vi "TIFF camera test 3.vi"(8 "Gain":i32=100 min=100 max=2000 step=1, 9 "Exposure time (ms)":dbl=100.0 min=1.0 max=10000.0 step=1.0) -> (2 "Image out":T1(plugin-control))   [LabVIEW 2017]
uses:
  libtiff/ctiff.llb/__CTIFFNewFileAndStyleUINT16.vi
  libtiff/ctiff.llb/__CTIFFAddNewPageUINT16.vi
panel:
  out "Saving":bool
  in  "delay (ms)":dbl=100.0 min=0.0 max=2000.0 step=1.0
  in  "#-frames":i32=100 min=0 max=2000 step=1
  out "Capturing":bool
  in  "TIF file path":path=path "C:/Users/Chip Scope/Desktop/test.tif"
  in  "stop":bool
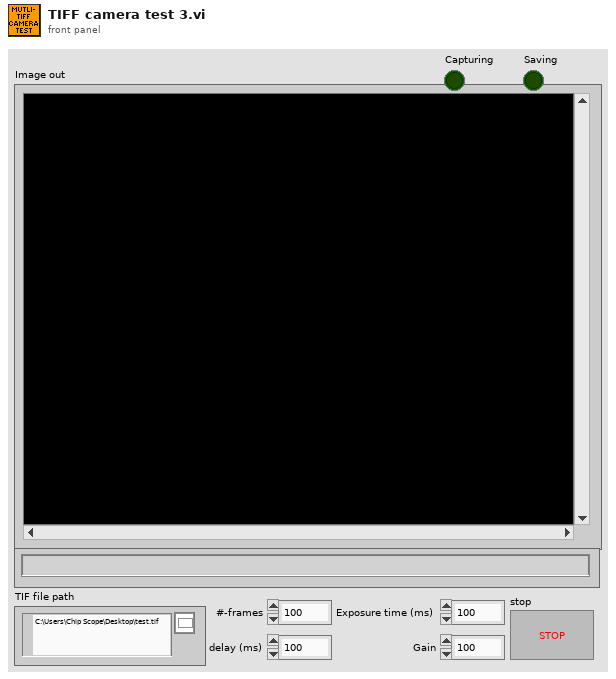
[diagram p1: front panel]
types:
  T1 = typedef "IMAQ Image.ctl" = refnum<image>
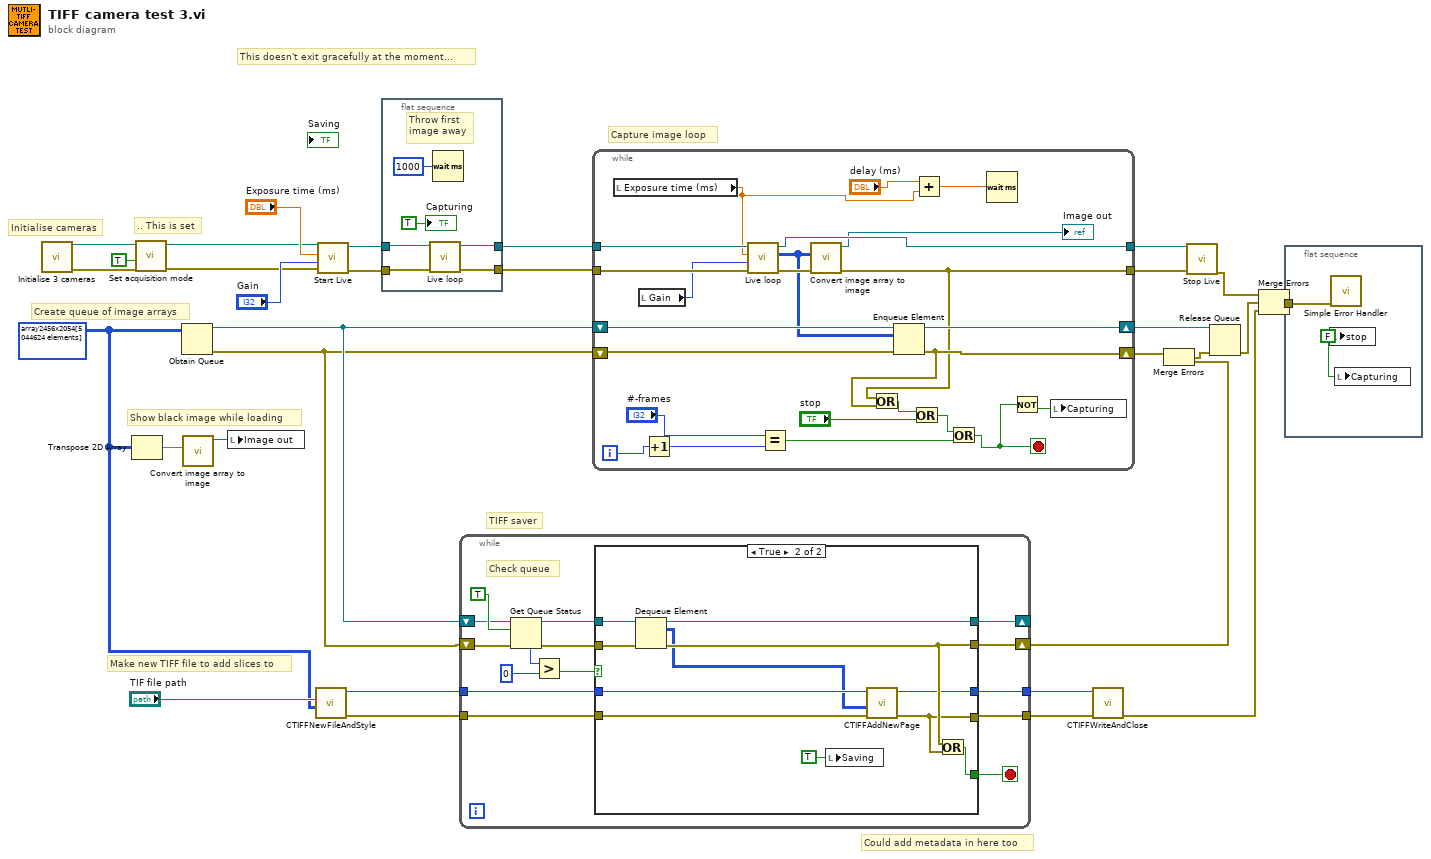
[diagram p0: block diagram]
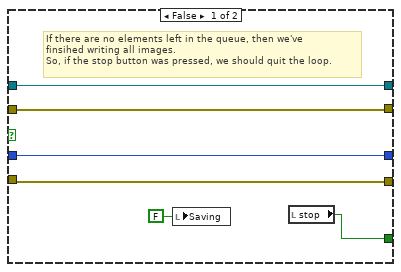
[diagram p2: hidden frame]
diagram:
  w12 = u16[][] array2456x2054[5044624 elements] ("Image Array")
  # ".. This is set"
  # "This doesn't exit gracefully at the moment..."
  # "Show black image while loading"
  # "Could add metadata in here too"
  # "Make new TIFF file to add slices to"
  # "Initialise cameras"
  # "Create queue of image arrays"
  # "TIFF saver"
  # "Capture image loop"
  n1 = call "Initialise 3 cameras.vi"() -> ("Error Out"=w8:errorcluster, "Red camera ref"=w9:refnum<k24>)  [unwired: 8 in, 2 out]
  n2 = Transpose 2D Array(2D array=w12) -> (transposed array=w11:u16[][])
  n3 = call "Set acquisition mode.vi"("Error In"=w8, "Synchronous acquisition"=TRUE, "Camera reference in"=w9) -> ("Error Out"=w7:errorcluster, "Camera reference out"=w6:refnum<k24>)  [unwired: 7 in]
  n4 = Obtain Queue(element data type=w12) -> (queue out=w23:refnum<queue>, error out=w22:errorcluster)  [unwired: 4 in, 1 out]
  n5 = call "Convert image array to image.vi"("Array"=w11) -> ("Image Out"=w10:T1)  [unwired: 8 in, 1 out]
  n6 = local write "Image out"(w10) -> ()
  n7 = call-poly "CTIFFNewFileAndStyle.vi"("image"=w12, "output_file"="TIF file path") -> ("error"=w16:errorcluster, "CTIFF"=w17:i64)  [unwired: 8 in]
  n8 = call "Start Live.vi"("Error In"=w7, "Gain in"="Gain", "Exposure time (ms)"="Exposure time (ms)", "Camera reference in"=w6) -> ("Error Out"=w4:errorcluster, "Camera reference out"=w2:refnum<k24>)  [unwired: 5 in]
  n9 = flat-sequence {
    tunnel: [w33] -> w3
    tunnel: w4 -> [w32]
    tunnel: w2 -> [w35]
    tunnel: [w34] -> w1
    frame #0 {
      # "Throw first\nimage away"
      n10 = call "Live loop.vi"("Error In"=w32, "Camera reference in"=w35) -> ("Error Out"=w33:errorcluster, "Camera reference out"=w34:refnum<k24>)  [unwired: 6 in, 1 out]
      n11 = Wait (ms)(milliseconds to wait=u32 1000) -> ()  [unwired: 1 out]
      "Capturing" <- TRUE ("Capturing")
    }
  }
  n12 = while {
    shift-right: [w52] -> _
    shift-left: w23 -> [w42]
    shift-right: [w50] -> w21
    shift-left: w22 -> [w45]
    tunnel: w17 -> [w41]
    tunnel: w16 -> [w40]
    tunnel: [w39] -> w15
    tunnel: [w38] -> w14
    stop <- w51 stop-if-true
    # "Check queue"
    n13 = Get Queue Status(queue=w42, return elements? (F)=TRUE, error in (no error)=w45) -> (queue out=w43:refnum<queue>, error out=w44:errorcluster, # elements in queue=w48:i32)  [unwired: 5 out]
    n14 = Greater?(x=w48, y=0) -> (0:w46:bool)
    n15 = case shown="True" w46 {
      tunnel: w43 -> [w58 w69]
      tunnel: w44 -> [w57 w68]
      tunnel: [w58 w67] -> w52
      tunnel: [w54 w66] -> w51
      tunnel: [w57 w65] -> w50
      tunnel: w41 -> [w56 w64]
      tunnel: w40 -> [w55 w63]
      tunnel: [w56 w62] -> w39
      tunnel: [w55 w61] -> w38
      frame False {
        # "If there are no elements left in the queue, then we've \nfinsihed writing all images. \nSo, if the stop button was pressed, we should quit the loop."
        n16 = local write "Saving"(FALSE ("Saving")) -> ()
        n17 = local read "stop"() -> (w54:bool)
      }
      frame True {
        n18 = Dequeue Element(queue=w69, error in (no error)=w68) -> (queue out=w67:refnum<queue>, element=w60:u16[][], error out=w65:errorcluster)  [unwired: 1 in, 1 out]
        n19 = local write "Saving"(TRUE ("Saving")) -> ()
        n20 = call-poly "CTIFFAddNewPage.vi"("error"=w63, "image"=w60, "CTIFF"=w64) -> ("error"=w61:errorcluster, "CTIFF"=w62:i64)  [unwired: 7 in]
        n21 = Or(x=w65, y=w61) -> (x .or. y?=w66:bool)
      }
    }
  }
  n22 = while {
    tunnel: [w81] -> w31
    tunnel: [w93] -> w30
    tunnel: w1 -> [w92]
    tunnel: w3 -> [w91]
    shift-right: [w85] -> w29
    shift-left: w23 -> [w87]
    shift-right: [w84] -> w27
    shift-left: w22 -> [w86]
    i -> [w73]
    stop <- w70 stop-if-true
    n23 = local read "Exposure time (ms)"() -> (w78:dbl)
    n24 = local read "Gain"() -> (w90:i32)
    n25 = Increment(x=w73) -> (x+1=w72:i32)
    n26 = call "Live loop.vi"("Error In"=w91, "Gain"=w90, "Exposure time (ms)"=w78, "Camera reference in"=w92) -> ("Error Out"=w82:errorcluster, "Image Array"=w80:u16[][], "Camera reference out"=w93:refnum<k24>)  [unwired: 4 in]
    n27 = Equal?(x="#-frames", y=w72) -> (x = y?=w74:bool)
    n28 = call "Convert image array to image.vi"("Error In"=w82, "Array"=w80) -> ("error out"=w81:errorcluster, "Image Out"=→"Image out":T1)  [unwired: 7 in]
    n29 = Enqueue Element(queue=w87, element=w80, error in (no error)=w86) -> (queue out=w85:refnum<queue>, error out=w84:errorcluster)  [unwired: 1 in, 1 out]
    n30 = Or(x=w81, y=w84) -> (x .or. y?=w89:bool)
    n31 = Or(x=w89, y="stop") -> (x .or. y?=w75:bool)
    n32 = Add(x="delay (ms)", y=w78) -> (x+y=w77:dbl)
    n33 = Or(x=w75, y=w74) -> (x .or. y?=w70:bool)
    n34 = Wait (ms)(milliseconds to wait=w77) -> ()  [unwired: 1 out]
    n35 = Not(x=w70) -> (.not. x?=w71:bool)
    n36 = local write "Capturing"(w71) -> ()
  }
  n37 = call "CTIFFWriteAndClose.vi"("error"=w14, "CTIFF"=w15) -> ("error"=w13:errorcluster)  [unwired: 9 in]
  n38 = Merge Errors(w27, w21) -> (w28:errorcluster)
  n39 = call "Stop Live.vi"("Camera reference in"=w30, "Error In"=w31) -> ("Error Out"=w26:errorcluster)  [unwired: 16 in, 1 out]
  n40 = Release Queue(queue=w29, error in (no error)=w28) -> (error out=w25:errorcluster)  [unwired: 1 in, 2 out]
  n41 = Merge Errors(w26, w25, w13) -> (w24:errorcluster)
  n42 = flat-sequence {
    tunnel: w24 -> [w95]
    frame #0 {
      w94 = FALSE ("stop")
      n43 = local write "stop"(w94) -> ()
      n44 = call <vilib>:"Simple Error Handler.vi"("error in (no error)"=w95) -> ()  [unwired: 4 in, 5 out]
      n45 = local write "Capturing"(w94) -> ()
    }
  }
